vi "Test 3 Serial Read Data is Written to Log.vi"(8 "error in (no error)":errorcluster, 11 "Test Case In":refnum<class "Serial Logging Decorator Test.lvclass">) -> (0 "error out":errorcluster, 3 "Test Case Out":refnum<class "Serial Logging Decorator Test.lvclass">)   [LabVIEW 2020, in "Serial Logging Decorator Test.lvclass"]
uses:
  Serial Logging Decorator Test.lvclass
  C:/Program Files (x86)/National Instruments/LabVIEW 2020/vi.lib/Astemes/LUnit/Test Case.lvclass
  Mock Serial/Mock Serial.lvclass
  C:/git/astemes-lmock/source/Examples/Serial Driver/Serial/Serial.lvclass/Serial.lvclass
  Log Mock/Mock Log.lvclass
  C:/git/astemes-lmock/source/Framework/Mock/LMock Mock.lvclass
  C:/git/astemes-lmock/source/Examples/Serial Driver/Log/Log.lvclass
  Serial/Serial.lvclass/Serial.lvclass
  Serial Logging Decorator Test.lvclass/Serial Logging Decorator Test.ctl
  Serial Logging Decorator/Serial Logging Decorator.lvclass
  Framework/LMock API.lvlib
  Framework/Verifier/Verifier.lvclass
  C:/git/astemes-lmock/source/Examples/Serial Driver/Log Mock/Mock Log.lvclass
  Expectations/One/One Matching String Inputs.vi
  Expectations/One/One.lvlib
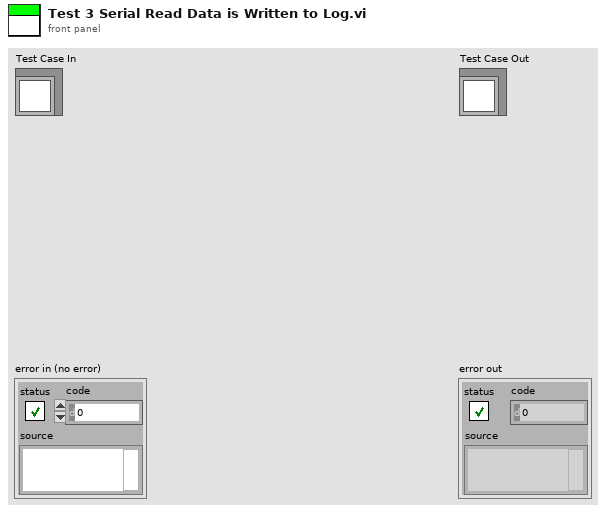
[diagram p1: front panel]
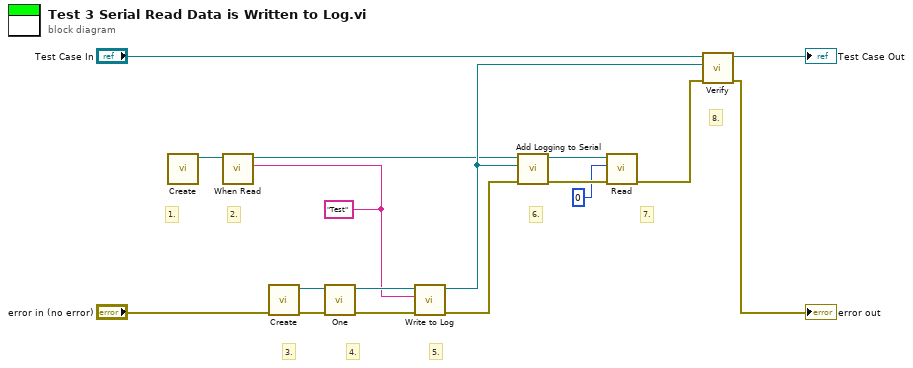
[diagram p0: block diagram]
diagram:
  w3 = "Test" ("Text to Write")
  # "8."
  # "7."
  # "6."
  # "5."
  # "4."
  # "3."
  # "2."
  # "1."
  n1 = call "Create.vi"() -> ("Mock Class Generator out"=w4:refnum<class "Mock Serial.lvclass">)  [unwired: 10 in, 1 out]
  n2 = call "When Read.vi"("read buffer"=w3, "Serial in"=w4) -> ("Serial out"=w2:refnum<class "Mock Serial.lvclass">)  [unwired: 9 in]
  n3 = call "Create.vi"("error in (no error)"="error in (no error)") -> ("error out"=w13:errorcluster, "Mock Class Generator out"=w14:refnum<class "Mock Log.lvclass">)  [unwired: 9 in]
  n4 = call-poly "One.vi"("error in (no error)"=w13, "Mock in"=w14) -> ("error out"=w11:errorcluster, "Mock out"=w12:refnum<class "Mock Log.lvclass">)  [unwired: 8 in]
  n5 = call-dynamic "Write to Log.vi"("error in (no error)"=w11, "Text to Write"=w3, "Log in"=w12) -> ("error out"=w8:errorcluster, "Log out"=w5:refnum<class "Mock Log.lvclass">)  [unwired: 7 in]
  n6 = call "Add Logging to Serial.vi"("error in (no error)"=w8, "Log Destination"=w5, "Serial"=w2) -> ("error out"=w9:errorcluster, "Serial with Logging"=w10:refnum<class "Serial.lvclass">)  [unwired: 7 in]
  n7 = call-dynamic "Read.vi"("error in (no error)"=w9, "byte count"=u32 0, "Serial in"=w10) -> ("error out"=w6:errorcluster)  [unwired: 6 in, 2 out]
  n8 = call "Verify.vi"("error in (no error)"=w6, "Mock"=w5, "LUnit Test Case In"="Test Case In") -> ("error out"=→"error out":errorcluster, "LUnit Test Case Out"=→"Test Case Out":refnum<class "Serial Logging Decorator Test.lvclass">)  [unwired: 7 in]
